vi "Unpack Value Change.vi"(11 "ValueChangeMsg In":refnum<class "ValueChangeMsg.lvclass">) -> (0 "New Value":variant, 1 "Old Value":variant, 2 "Time":u32, 3 "Name":string)   [LabVIEW 2015, in "ActorAutoRegistration.lvlib" / "ValueChangeMsg.lvclass"]
doc: "<License>\nCopyright © 2017 Composed Systems, LLC | All rights reserved\nwww.composed.io\n\nAuthor: Ethan Stern <ethan.stern@composed.io>\n\nThis software is provided \"AS IS\" WITHOUT WARRANTIES, either express or implied, AND IS FOR EDUCATIONAL PURPOSES ONLY.\n</License>"
uses:
  ValueChangeMsg.lvclass
  ValueChangeMsg.lvclass/ValueChangeMsg.ctl
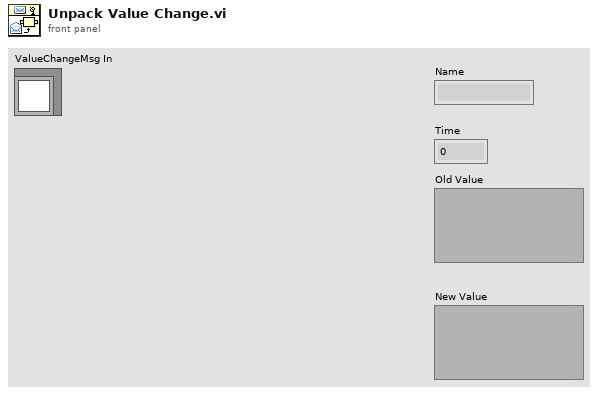
[diagram p1: front panel]
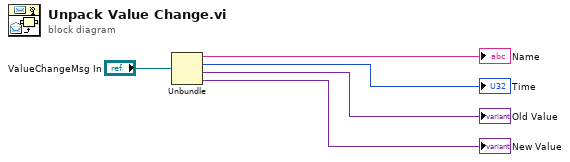
[diagram p0: block diagram]
diagram:
  n1 = Unbundle("ValueChangeMsg In") -> (→"Name":string, →"Time":u32, →"Old Value":variant, →"New Value":variant)
